vi "Triangle process.vi"(0 "error in":errorcluster) -> ()   [LabVIEW 2012]
uses:
  Triangle global info.vi
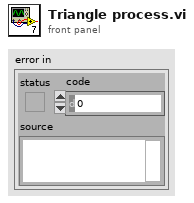
[diagram p1: front panel]
types:
  T1 = cluster{"Button 6":bool, "Button 7":bool, "Button 10":bool, "Button 11":bool, "Triangles values":dbl[]}
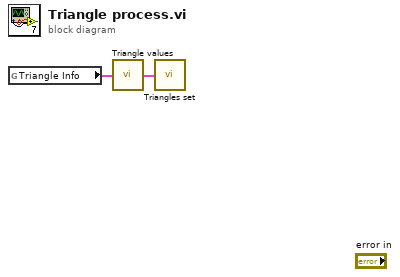
[diagram p0: block diagram]
diagram:
  n1 = global read "Triangle global info.vi" "Triangle Info"() -> (w1:T1)
  n2 = call "Triangle values.vi"("Triangle Info"=w1) -> ("Triangle Info Out"=w2:T1)
  n3 = call "Triangles set.vi"("Triangle Info"=w2) -> ()
